vi "Configure Level.vi"(4 "attenuation":dbl caption="attenuation (dB)", 5 "attenuation auto (Off)":bool, 6 "reference level offset":dbl, 7 "reference level":dbl, 8 "error in (no error)":errorcluster {"code" format="%.0x"}, 9 "input impedance":dbl, 10 "amplitude units (dBm)":i32(ring)=1 items=["dBm"=1, "dBmV"=2, "dBuV"=3, "Volt"=4, "Watt"=5], 11 "instrument handle":refnum<k15>) -> (0 "error out":errorcluster {"code" format="%.0x"}, 3 "instrument handle out":refnum<k15>)   [LabVIEW 2009, in "Keysight XSAn.lvlib"]
doc: "This VI configures the vertical properties of the IviSpecAn.\n\nSupported Models: M9290A, N8973B, N8974B, N8975B, N8976B, N9000A, N9000B, N9010A, N9010B, N9020A, N9020B, N9030A, N9030B, N9038A, N9040B, N9041B, SPN9003A, SPN9026A"
uses:
  <instrlib>/Keysight XSAn/Keysight XSAn.lvlib
  AgXSAn.dll
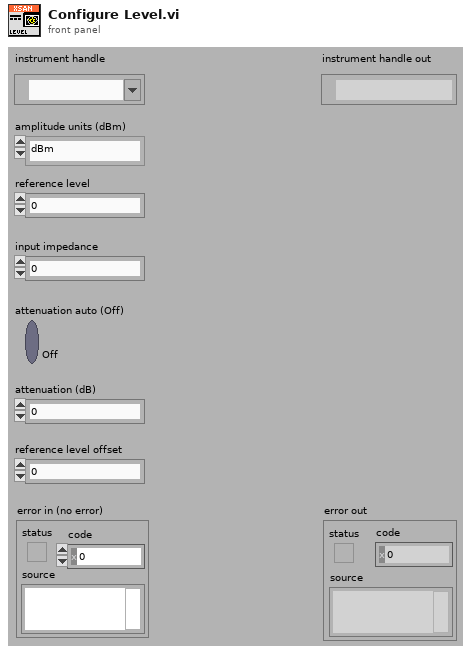
[diagram p1: front panel]
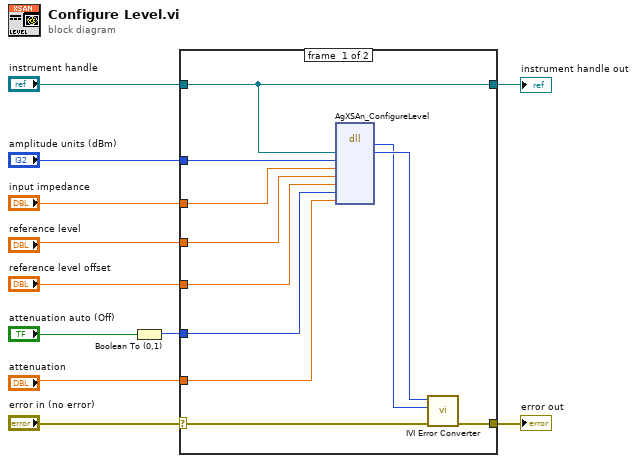
[diagram p0: block diagram]
diagram:
  n1 = Boolean To (0,1)(Boolean="attenuation auto (Off)") -> (0, 1=w2:i16)
  n2 = case shown="No Error" "error in (no error)" {
    selector: "error in (no error)" -> [w20 w24]
    tunnel: [w21 w24] -> w10
    tunnel: "instrument handle" -> [w18 w23]
    tunnel: [w18 w23] -> w8
    tunnel: "amplitude units (dBm)" -> [w17 _]
    tunnel: "input impedance" -> [w16 _]
    tunnel: "reference level" -> [w15 _]
    tunnel: "reference level offset" -> [w14 _]
    tunnel: w2 -> [w12 _]
    tunnel: "attenuation" -> [w13 _]
    frame #0 {
      n3 = dll-call lib="AgXSAn**.dll" fn="AgXSAn_ConfigureLevel" ("LabVIEW:IviSpecAn_ConfigureLevel")("instrument handle"=w18, "amplitude units"=w17, "input impedance"=w16, "reference level"=w15, "reference level offset"=w14, "attenuation auto"=w12, "attenuation"=w13) -> ("Status"=w19:i32, "instrument handle"=w22:u32)  [unwired: 9 in, 2 out]
      n4 = call <instrlib>:"IVI Error Converter.vi"("error in (no error)"=w20, "IVI error code (0)"=w19, "instrument handle"=w22) -> ("error out"=w21:errorcluster)  [unwired: 7 in, 1 out]
    }
    frame #1 {
    }
  }
  "error out" <- w10
  "instrument handle out" <- w8
